vi "Cobra Launch.vi"() -> ()   [LabVIEW 2019]
uses:
  Cobra/Cobra/Cobra.lvclass
  C:/Program Files (x86)/National Instruments/LabVIEW 2019/vi.lib/ActorFramework/Actor/Actor.lvclass
  <vilib>/NI/Actors/Network Endpoint Actors/Protocols/Network Stream Strategy/Network Stream/Network Stream.lvclass/Network Stream.ctl
  <vilib>/ni/Actors/Network Endpoint Actors/Protocols/Network Stream Strategy/Network Stream Initiator/Network Stream Initiator.lvclass/Network Stream Initiator.ctl
  Cobra/Cobra/Cobra.lvclass/Cobra.ctl
  <vilib>/NI/Actors/Network Endpoint Actors/Protocols/Network Stream Strategy/Network Stream/Write Buffer Size.vi
  <vilib>/NI/Actors/Network Endpoint Actors/Protocols/Network Stream Strategy/Network Stream/Write Name.vi
  <vilib>/ni/Actors/Network Endpoint Actors/Protocols/Network Stream Strategy/Network Stream Initiator/Network Stream Initiator.lvclass
  C:/Program Files (x86)/National Instruments/LabVIEW 2019/vi.lib/NI/Actors/Network Endpoint Actors/Protocols/Network Stream Strategy/Network Stream/Network Stream.lvclass
  C:/Program Files (x86)/National Instruments/LabVIEW 2019/vi.lib/NI/Actors/Network Endpoint Actors/Abstract Classes/Message Stream/Message Stream.lvclass
  <vilib>/ActorFramework/Actor/Actor.lvclass
panel:
  in  "Listener Name":string="Bob"
  in  "Address":string="127.0.0.1"
  in  "Initiator Name":string="Fred"
  out "error out":errorcluster
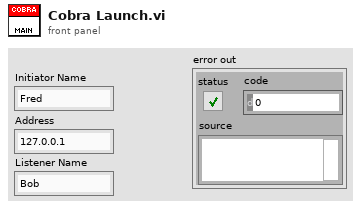
[diagram p1: front panel]
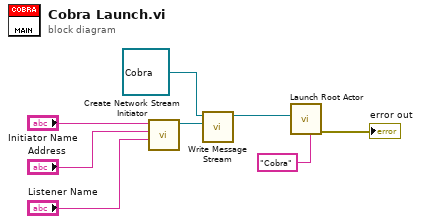
[diagram p0: block diagram]
diagram:
  n1 = call <vilib>:"Create Network Stream Initiator.vi"("Remote Name"="Listener Name", "Remote Address"="Address", "Name"="Initiator Name") -> ("Network Stream Initiator out"=w3:refnum<class "Network Stream Initiator.lvclass">)  [unwired: 8 in]
  n2 = call "Write Message Stream.vi"("Message Stream"=w3, "Cobra In"=refnum<class "Cobra.lvclass"> refnum ("Cobra.lvlib:Cobra.lvclass")) -> ("Cobra out"=w1:refnum<class "Cobra.lvclass">)  [unwired: 9 in]
  n3 = call <vilib>:"Launch Root Actor.vi"("Debug Alias"="Cobra", "Actor"=w1) -> ("error out"=→"error out":errorcluster)  [unwired: 8 in, 1 out]
